vi "Global communication output.vi"() -> ()   [LabVIEW 2016]
panel:
  in  "Analog output":dbl[](array[numeric])
  in  "Matrix output":bool
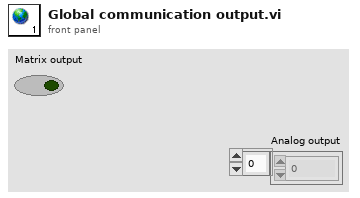
[diagram p1: front panel]
diagram:
